vi "3_AdvancedDemo_MHT3.vi"() -> ()   [LabVIEW 2010]
uses:
  Types/MH_UIThread_Cmds.ctl
  _lib/PQ/MultiHarp/MH_InitInfo.ctl
  Types/MH_UIThread_Data.ctl
  Types/MH_InputChannel.ctl
  _lib/PQ/MultiHarp/MH_RefSource.ctl
  _lib/PQ/MultiHarp/mhlib_x86_x64_UIThread.llb/MH_DllPath_global.vi
  <vilib>/Utility/error.llb/DialogType.ctl
  Types/MH_DataProcThread_QCmds.ctl
  Types/MH_DataProcThread_QData.ctl
  Types/MH_VisThread_QCmds.ctl
  Types/MH_VisThread_QData.ctl
  Types/MH_VisThread_Data.ctl
  _lib/PQ/MultiHarp/MH_LibVersion_global.vi
  _lib/PQ/MultiHarp/MH_MeasMode.ctl
  Types/MH_SetInpChanData.ctl
  Types/MH_SetInpChanCmds.ctl
panel:
  in  "Settings":bool=TRUE
  in  "Run continuously":bool caption="Conti."
  in  "Start":bool
  in  "Scale":bool
  out "CountRates":i32[](graph)
  in  "AllChannels":T1={"Enable"=TRUE, "Offset"=0, "Level"=-100, "Edge"=0, "DeadTime"=1000, "UseDeadTime"=FALSE, "SetEnableAllChan"=TRUE, "SetEdgeAllChan"=TRUE, "SetLevelAllChan"=TRUE, "SetOffsetAllChan"=TRUE, "SetUseDTAllChan"=TRUE, "SetDeadTAllChan"=TRUE} {"DeadTime" min=800 max=160000 step=1; "Edge" items=["falling", "rising"]; "Offset" min=-100000 max=100000 step=80; "Level" min=-1200 max=1200 step=1}
  in  "HistoAcqTime":dbl=1.0 caption="Hist.Int.Time  s" min=0.1 max=360000.0 step=0.1
  in  "AcqTime":i32=360000000 caption="T3Acqu.       ms" min=1 max=360000 step=1
  in  "Binning":i32(ring) caption="Resol.            ps" items=["80", "160", "320", "640", "1280", "2560", "5120", "10240", "20480", "40960", "81920", "163840", "327680", "655360", "1310720", "2621440", "5242880", "10485760", "20971520", "41943040", "83886080", "167772160", "335544320"]
  in  "HistoOffset":i32 caption="Offset            ns" min=0 max=100000000 step=1
  out "DeltaT":dbl=6.553665536655367 caption="T.Tr.Resol.   ms" format="%.2f"
  in  "BitShift":i32=15 min=0 max=32 step=1
  in  "OvlLevel":u32=4294967295 caption="Ovl.Level" min=1024 max=65536 step=1024
  in  "StopOvl.":bool=TRUE
  out "TTraceGraph":T2(graph)={49.38852226226715, "Resolution"=0.00655367864414373, "Histogram"=[]}
  out "HistoGraph":cluster{dbl, "Resol":dbl, "Histos":u32[][]}(graph)={0.0, "Resol"=0.08, "Histos"=[]}
  in  "SyncDeadTime":i32=1000 caption="Dead T.   ps" min=800 max=160000 step=1
  in  "UseDeadTime":bool caption="Use DT."
  in  "SyncEdge":i32(ring) caption="Edge" items=["falling", "rising"]
  in  "SyncDivider":i32(ring) caption="Divider" items=["1", "2", "4", "8", "16"]
  in  "SyncOffset":i32 caption="Offset      ps" min=-100000 max=100000 step=80
  in  "SyncLevel":i32=-100 caption="Level      mV" min=-1200 max=1200 step=1
  in  "Channels":T3[](array[typedef])=[{"Name"="Inp.Chan 1", "Enable"=TRUE, "Edge"=0, "Level"=-100, "Offset"=0, "UseDeadTime"=FALSE, "DeadTime"=1000}, {"Name"="Inp.Chan 2", "Enable"=TRUE, "Edge"=0, "Level"=-100, "Offset"=0, "UseDeadTime"=FALSE, "DeadTime"=1000}, {"Name"="Inp.Chan 3", "Enable"=TRUE, "Edge"=0, "Level"=-100, "Offset"=0, "UseDeadTime"=FALSE, "DeadTime"=1000}, {"Name"="Inp.Chan 4", "Enable"=TRUE, "Edge"=0, "Level"=-100, "Offset"=0, "UseDeadTime"=FALSE, "DeadTime"=1000}, {"Name"="Inp.Chan 5", "Enable"=TRUE, "Edge"=0, "Level"=-100, "Offset"=0, "UseDeadTime"=FALSE, "DeadTime"=1000}, {"Name"="Inp.Chan 6", "Enable"=TRUE, "Edge"=0, "Level"=-100, "Offset"=0, "UseDeadTime"=FALSE, "DeadTime"=1000}, {"Name"="Inp.Chan 7", "Enable"=TRUE, "Edge"=0, "Level"=-100, "Offset"=0, "UseDeadTime"=FALSE, "DeadTime"=1000}, {"Name"="Inp.Chan 8", "Enable"=TRUE, "Edge"=0, "Level"=-100, "Offset"=0, "UseDeadTime"=FALSE, "DeadTime"=1000}, {"Name"="Inp.Chan 9", "Enable"=TRUE, "Edge"=0, "Level"=-100, "Offset"=0, "UseDeadTime"=FALSE, "DeadTime"=1000}, {"Name"="Inp.Chan 10", "Enable"=TRUE, "Edge"=0, "Level"=-100, "Offset"=0, "UseDeadTime"=FALSE, "DeadTime"=1000}, {"Name"="Inp.Chan 11", "Enable"=TRUE, "Edge"=0, "Level"=-100, "Offset"=0, "UseDeadTime"=FALSE, "DeadTime"=1000}, {"Name"="Inp.Chan 12", "Enable"=TRUE, "Edge"=0, "Level"=-100, "Offset"=0, "UseDeadTime"=FALSE, "DeadTime"=1000}, {"Name"="Inp.Chan 13", "Enable"=TRUE, "Edge"=0, "Level"=-100, "Offset"=0, "UseDeadTime"=FALSE, "DeadTime"=1000}, {"Name"="Inp.Chan 14", "Enable"=TRUE, "Edge"=0, "Level"=-100, "Offset"=0, "UseDeadTime"=FALSE, "DeadTime"=1000}, {"Name"="Inp.Chan 15", "Enable"=TRUE, "Edge"=0, "Level"=-100, "Offset"=0, "UseDeadTime"=FALSE, "DeadTime"=1000}, {"Name"="Inp.Chan 16", "Enable"=TRUE, "Edge"=0, "Level"=-100, "Offset"=0, "UseDeadTime"=FALSE, "DeadTime"=1000}] {"DeadTime" min=800 max=160000 step=1; "Edge" items=["falling", "rising"]; "Offset" min=-100000 max=100000 step=80; "Level" min=-1200 max=1200 step=1}
  out "SyncRate":string="Sync Rate: 4999940 cps\n"
  out "OverRun":bool caption="Overrun:"
  out "Status":string="Elements in Q: 0"
  # "All Channels"
  # "Acquisition"
  # "Sync"
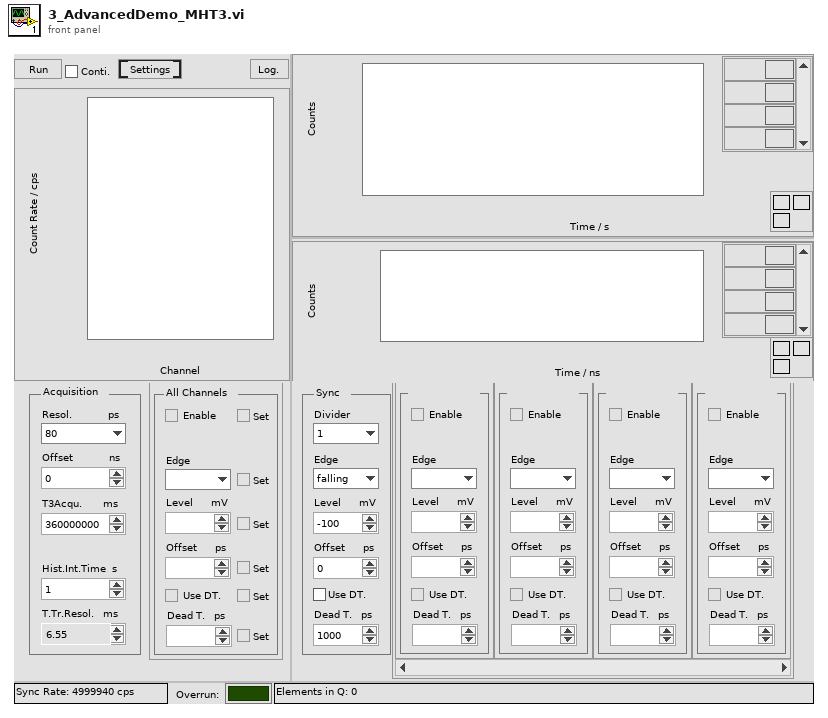
[diagram p1: front panel]
types:
  T1 = cluster{"Enable":bool, "Offset":i32, "Level":i32, "Edge":i32, "DeadTime":i32, "UseDeadTime":bool, "SetEnableAllChan":bool, "SetEdgeAllChan":bool, "SetLevelAllChan":bool, "SetOffsetAllChan":bool, "SetUseDTAllChan":bool, "SetDeadTAllChan":bool}
  T2 = cluster{dbl, "Resolution":dbl, "Histogram":u32[][]}
  T3 = typedef "MH_InputChannel.ctl" = cluster{"Name":string, "Enable":bool, "Edge":i32, "Level":i32, "Offset":i32, "UseDeadTime":bool, "DeadTime":i32}
  T4 = typedef "MH_DataProcThread_QCmds.ctl" = enum16{"Exit", "Proc", "Init", "SetShift", "SetNumChannels", "SetHistAcqTime"}
  T5 = typedef "MH_VisThread_Data.ctl" = cluster{"Resol":dbl, "DeltaT":dbl, "NumChannels":i32}
  T6 = typedef "MH_VisThread_QData.ctl" = cluster{"Histos":u32[][], "Cmd":T7, "TimeTrace":u32[][], "Bin":i32, "Total bin":u64, "Status":string, "Resol":dbl, "DeltaT":dbl, "nChannels":i32}
  T7 = typedef "MH_VisThread_QCmds.ctl" = enum16{"_none_", "Resol", "nChannels", "DeltaT", "Histo", "TTrace", "Status"}
  T8 = typedef "MH_DataProcThread_QData.ctl" = cluster{"Cmd":T4, "nActual":i32, "Buffer":u32[], "TickCount":u32, "Param":i32}
  T9 = typedef "MH_UIThread_Data.ctl" = cluster{"Init Info":T10, "DevIdx":i32, "SyncDivider":i32, "SyncOffset":i32, "SyncLevel":i32, "Channels":T3[], "CurrentChannels":i32[], "AcqTime":i32, "Binning":i32, "HistoOffset":i32, "HistoLen":i32, "StopOvl.":bool, "OvlLevel":u32, "SyncEdge":i32, "StartMeas":bool, "HistoLength":i32, "Resolution":dbl, "Run cont.":bool, "Status":string, "SyncRate":i32, "BitShift":i32, "HistoAcqTime":dbl, "SyncRateStart":i32, "UseDeadTime":bool, "SyncDeadTime":i32, "SetInpChan":T11[]}
  T10 = typedef "MH_InitInfo.ctl" = cluster{"Library Version":string, "Serial No.":string, "Model":string, "Partnum":string, "Version":string, "features":i32, "nchannels":i32, "Base Resolution":dbl, "Bin Steps":i32}
  T11 = typedef "MH_SetInpChanData.ctl" = cluster{"Channel":i32, "Cmds":T12[], "Changed":cluster{"Name":bool, "Enable":bool, "Edge":bool, "Level":bool, "Offset":bool, "UseDeadTime":bool, "DeadTime":bool}}
  T12 = typedef "MH_SetInpChanCmds.ctl" = enum16{"SetInpChanEnable", "SetInpChanOffset", "SetInpChanDeadTime", "SetInpChanTrg"}
  T13 = typedef "MH_UIThread_Cmds.ctl" = enum16{"Idle", "Init", "SetInpChan", "SetSyncDivider", "SetSyncTrg", "SetSyncOffset", "SetSyncDeadTime", "SetBinning", "SetHistoOffset", "SetHistoLen", "SetStopOvl", "SetBitShift", "SetHistoAcqTime", "GetRates", "GetAllRates", "StartMeas", "StopMeas", "AbortMeas", "GetResolution", "GetHistos", "GetAllHistos", "ReadFiFo", "WriteStatus", "Resize", "EnableControls", "DisableControls", "Error", "Exit"}
  T14 = enum8{"Enabled", "Disabled", "Disabled and Grayed Out"}
  T15 = cluster{"[0]":bool, "[1]":bool, "[2]":bool, "[3]":bool, "[4]":bool, "[5]":bool}
  T16 = typedef "MH_MeasMode.ctl" = i32
  T17 = typedef "MH_RefSource.ctl" = enum16{"INTERNAL", "EXTERNAL_10MHZ", "WR_MASTER_GENERIC", "WR_SLAVE_GENERIC", "WR_GRANDM_GENERIC", "EXTN_GPS_PPS", "EXTN_GPS_PPS_UART", "WR_MASTER_MHARP", "WR_SLAVE_MHARP", "WR_GRANDM_MHARP"}
  T18 = typedef "DialogType.ctl" = u16
  T19 = cluster{"T0":dbl, "dt":dbl, "TimeTrace_out":u32[][]}
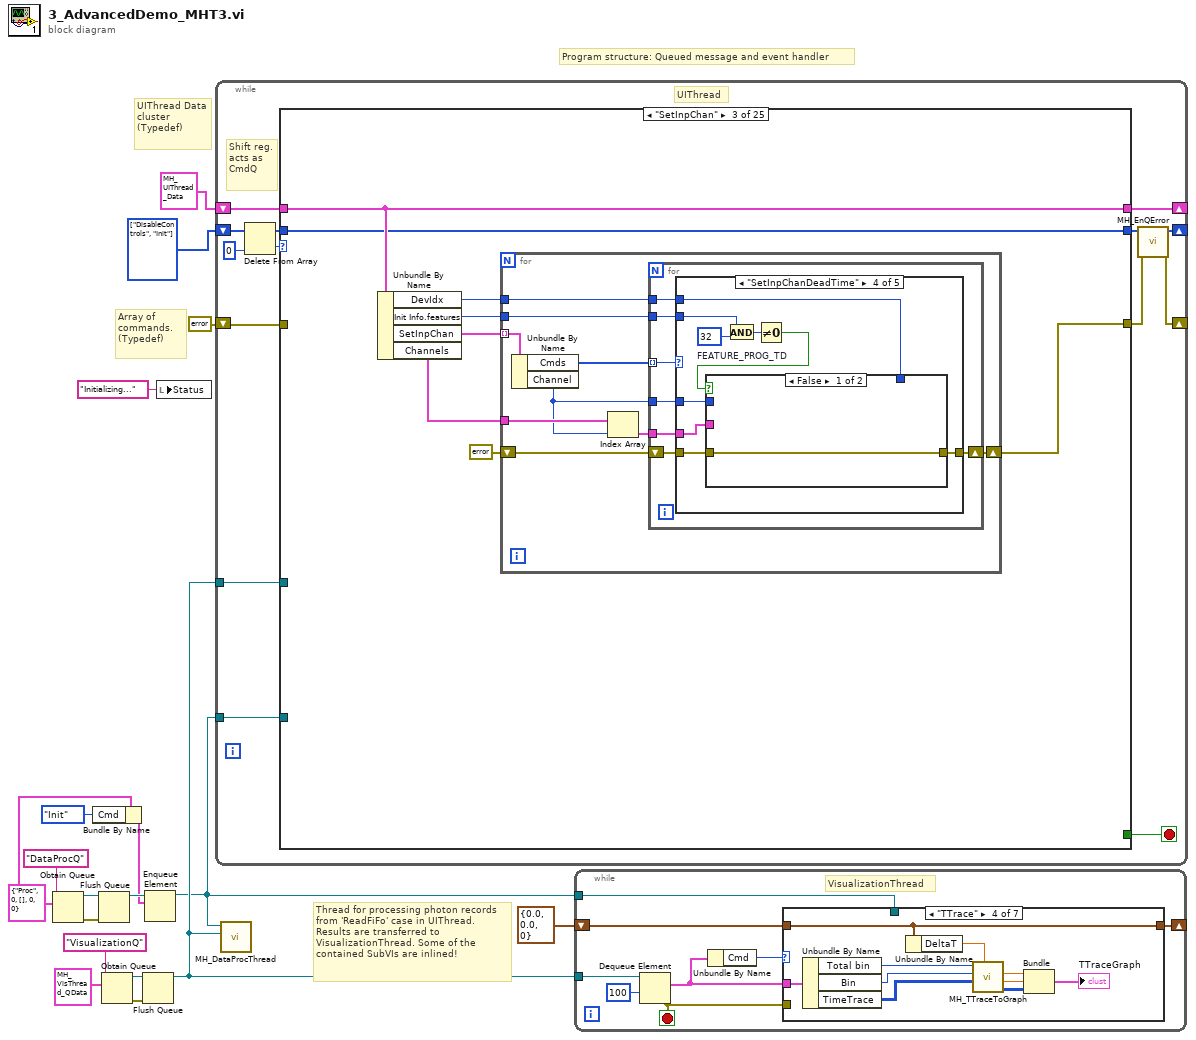
[diagram p0: block diagram]
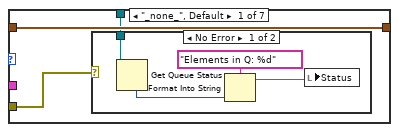
[diagram p2: hidden frame]
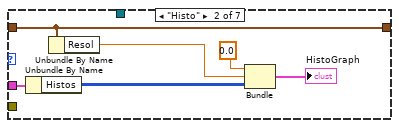
[diagram p4: hidden frame]
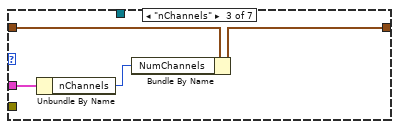
[diagram p5: hidden frame]
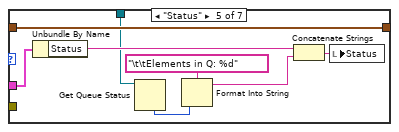
[diagram p6: hidden frame]
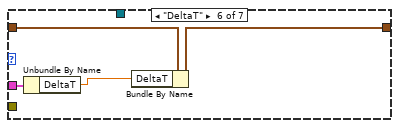
[diagram p7: hidden frame]
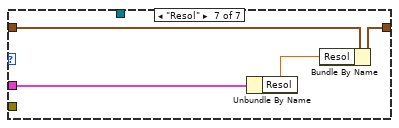
[diagram p8: hidden frame]
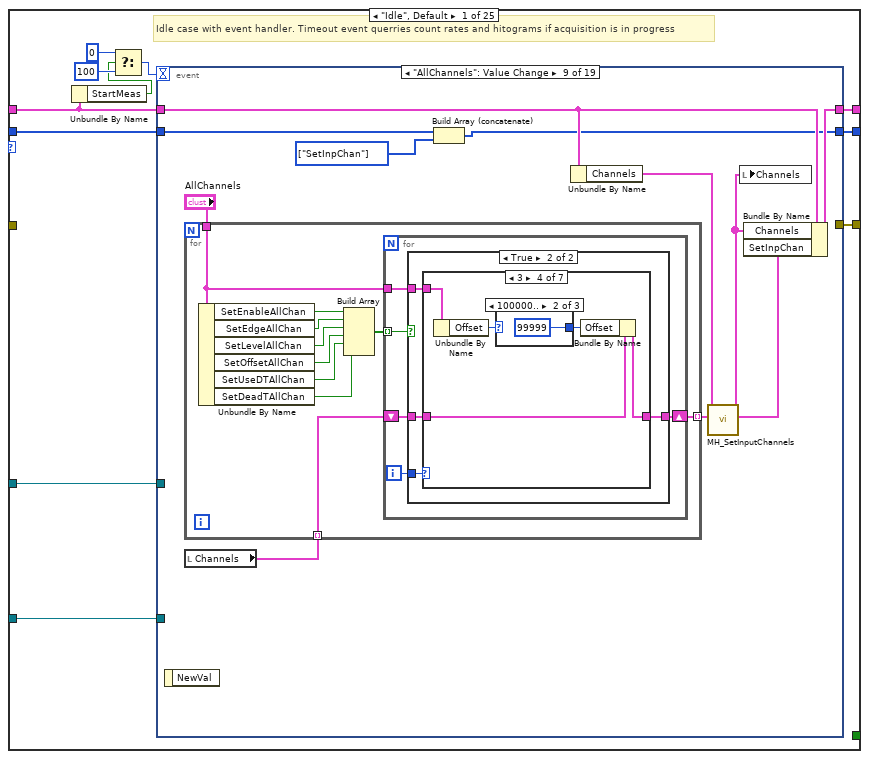
[diagram p9: hidden frame]
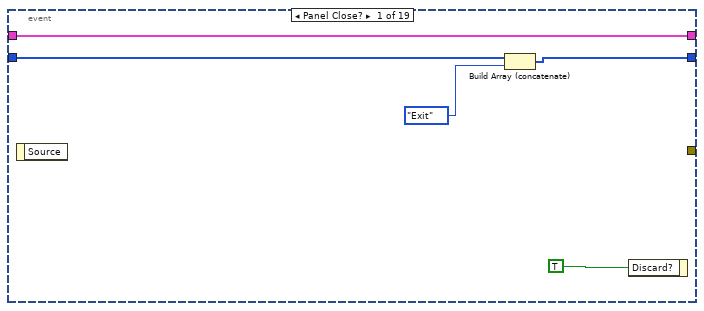
[diagram p10: hidden frame]
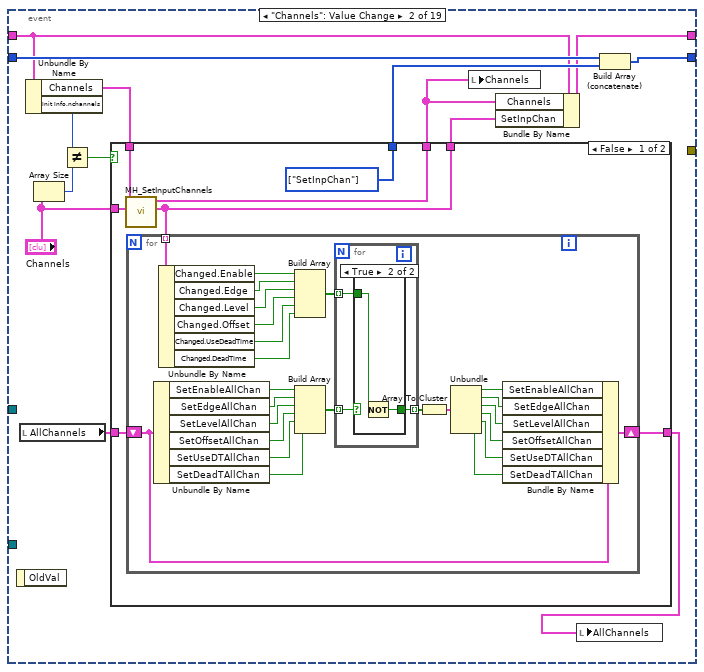
[diagram p11: hidden frame]
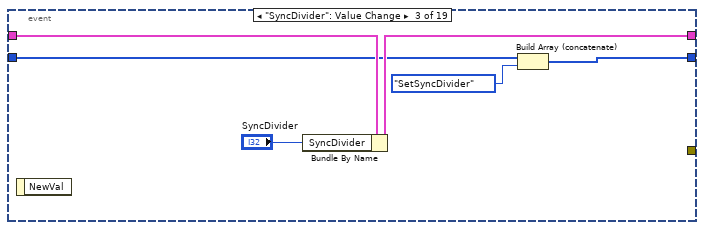
[diagram p14: hidden frame]
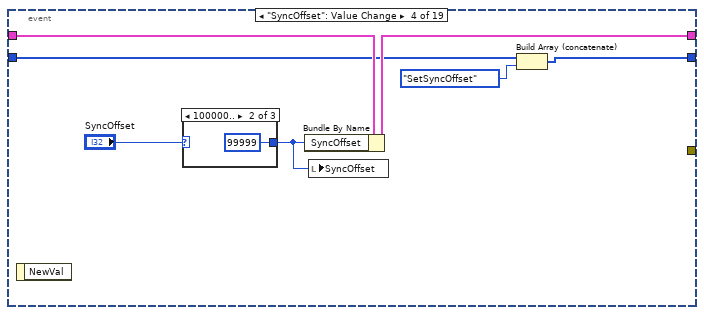
[diagram p15: hidden frame]
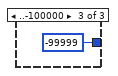
[diagram p17: hidden frame]
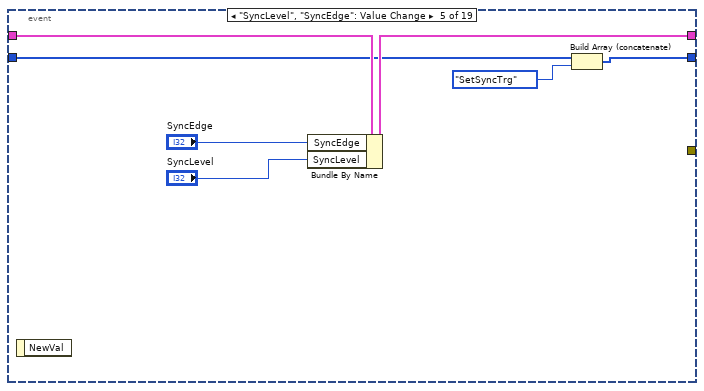
[diagram p18: hidden frame]
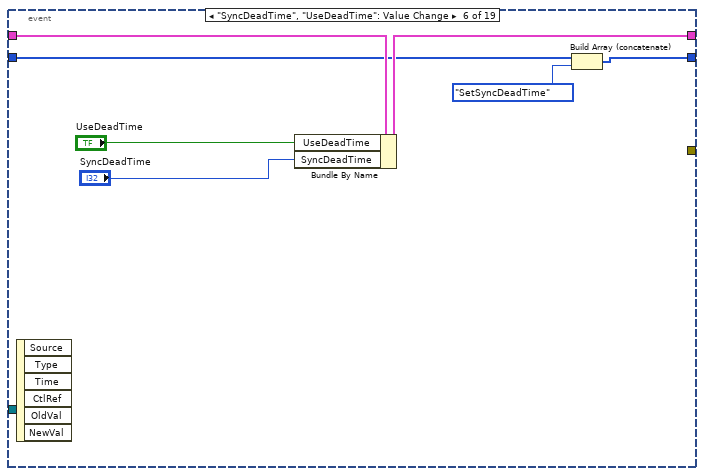
[diagram p19: hidden frame]
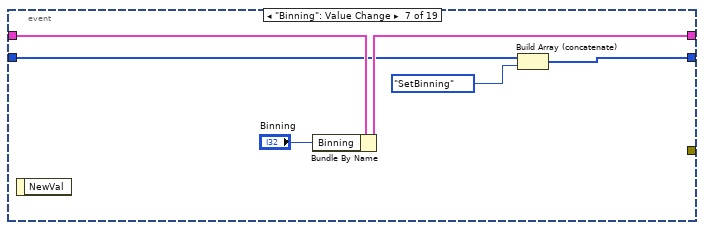
[diagram p20: hidden frame]
diagram:
  w4 = T8 {"Cmd"=enum."Proc", "nActual"=0, "Buffer"=[], "TickCount"=0, "Param"=0} ("MH_DataProcThread_QData")
  w17 = T13[] [enum."DisableControls", enum."Init"] items=["Idle", "Init", "SetInpChan", "SetSyncDivider", "SetSyncTrg", "SetSyncOffset", "SetSyncDeadTime", "SetBinning", "SetHistoOffset", "SetHistoLen", "SetStopOvl", "SetBitShift", "SetHistoAcqTime", "GetRates", "GetAllRates", "StartMeas", "StopMeas", "AbortMeas", "GetResolution", "GetHistos", "GetAllHistos", "ReadFiFo", "WriteStatus", "Resize", "EnableControls", "DisableControls", "Error", "Exit"]
  # "Thread for processing photon records from 'ReadFiFo' case in UIThread. Results are transferred to VisualizationThread. Some of the contained SubVIs are inlined!"
  # "Array of commands.\n(Typedef)"
  # "Program structure: Queued message and event handler"
  # "UIThread Data cluster\n(Typedef)"
  n1 = Obtain Queue(name (unnamed)="DataProcQ", element data type=w4) -> (queue out=w14:refnum<queue>, error out=w13:errorcluster)  [unwired: 3 in, 1 out]
  n2 = Bundle By Name(cluster=w4, "Cmd"=MH_DataProcThread_QCmds."Init") -> (w2:T8)
  n3 = Flush Queue(queue=w14, error in (no error)=w13) -> (queue out=w5:refnum<queue>)  [unwired: 2 out]
  n4 = Obtain Queue(name (unnamed)="VisualizationQ", element data type=T6 {"Histos"=[], "Cmd"=enum."_none_", "TimeTrace"=[], "Bin"=0, "Total bin"=0, "Status"="", "Resol"=0.0, "DeltaT"=0.0, "nChannels"=0} ("MH_GUIThread_QData")) -> (queue out=w12:refnum<queue>, error out=w11:errorcluster)  [unwired: 3 in, 1 out]
  n5 = Flush Queue(queue=w12, error in (no error)=w11) -> (queue out=w7:refnum<queue>)  [unwired: 2 out]
  n6 = Enqueue Element(queue=w5, element=w2) -> (queue out=w1:refnum<queue>)  [unwired: 2 in, 2 out]
  n7 = local write "Status"("Initializing..." ("Status")) -> ()
  n8 = while {
    shift-right: [w21] -> _
    shift-left: w17 -> [w28]
    shift-right: [w31] -> _
    shift-left: T9 {"Init Info"={"Library Version"="", "Serial No."="", "Model"="", "Partnum"="", "Version"="", "features"=0, "nchannels"=0, "Base Resolution"=0.0, "Bin Steps"=0}, "DevIdx"=0, "SyncDivider"=1, "SyncOffset"=0, "SyncLevel"=50, "Channels"=[], "CurrentChannels"=[], "AcqTime"=1, "Binning"=1, "HistoOffset"=1, "HistoLen"=1024, "StopOvl."=FALSE, "OvlLevel"=1024, "SyncEdge"=10, "StartMeas"=FALSE, "HistoLength"=0, "Resolution"=0.0, "Run cont."=FALSE, "Status"="", "SyncRate"=0, "BitShift"=0, "HistoAcqTime"=0.0, "SyncRateStart"=0, "UseDeadTime"=FALSE, "SyncDeadTime"=800, "SetInpChan"=[]} -> [w30]
    shift-right: [w23] -> _
    shift-left: errorcluster {"status"=FALSE, "code"=0, "source"=""} ("error IO") -> [w29]
    tunnel: w1 -> [w20]
    tunnel: w7 -> [w19]
    stop <- w32 stop-if-true
    # "Shift reg.\nacts as\nCmdQ"
    # "UIThread"
    n9 = Delete From Array(array=w28, index=0) -> (deleted portion=w26:T13, array with subset deleted=w25:T13[])  [unwired: 1 in]
    n10 = case shown="\"SetInpChan\"" w26 {
      tunnel: [w43 w357 w375 w437 w446 w458 w464 w471 w479 w486 w506 w518 w521 w593 w616 w621 w634 w651 w652 w678 w691 w698 w710 w716 w722] -> w22
      tunnel: [_ _ _ _ _ _ _ _ _ _ _ _ _ _ _ _ _ _ _ _ _ _ _ _ TRUE] -> w32
      tunnel: [w42 w338 w376 w439 w447 w459 w468 w475 w480 w487 w491 w508 w530 w585 w608 w624 w636 w647 w662 w677 w679 w697 w709 w717 w725] -> w31
      tunnel: w30 -> [w39 w343 w376 w439 w447 w459 w468 w475 w480 w487 w491 w508 w520 w586 w609 w625 w637 w648 w662 w677 w679 w697 w709 w717 w725]
      tunnel: [w40 w360 w370 w435 w445 w457 w467 w474 w478 w485 _ _ w526 w592 w619 w627 w639 w649 w657 _ _ _ _ _ w723] -> w24
      tunnel: w29 -> [_ _ _ _ _ _ _ _ _ _ _ _ _ _ _ _ _ _ _ _ _ _ _ w718 _]
      tunnel: w25 -> [w41 w359 w375 w437 w446 w458 w464 w470 w479 w486 w506 w518 w522 w593 w617 w622 w634 w651 w653 w678 w691 w698 w710 _ w722]
      tunnel: w20 -> [w34 w336 _ _ _ _ _ _ _ _ w492 w509 _ _ w613 _ _ _ w654 _ _ _ _ _ w721]
      tunnel: w19 -> [w33 w329 _ _ _ _ _ _ _ _ w493 _ _ _ _ _ _ w644 _ _ _ _ _ _ w720]
      frame "Idle", Default {
        # "Idle case with event handler. Timeout event querries count rates and hitograms if acquisition is in progress"
        n11 = Unbundle By Name(w39) -> ("StartMeas"=w37:bool)
        n12 = Select(t=0, s=w37, f=100) -> (s? t:f=w36:i32)
        n13 = event shown="[8] \"AllChannels\": Value Change" {
          selector: _ -> [_ _ _ _ _ _ _ _ _ _ _ _ _ _ _ _ _ _ _]
          dyn-events: _ -> [_ _ _ _ _ _ _ _ _ _ _ _ _ _ _ _ _ _ _]
          timeout: w36 -> [_ _ _ _ _ _ _ _ _ _ _ _ _ _ _ _ _ _ _]
          tunnel: [w44 w61 w103 w111 w120 w128 w134 w140 w145 w205 w210 w217 w232 w250 w262 w280 w286 w294 w304] -> w43
          tunnel: [w47 w53 w107 w114 w124 w131 w137 w143 w150 w207 w213 w220 w231 w254 w261 w278 w285 w293 w307] -> w42
          tunnel: w39 -> [w47 w54 w108 w115 w125 w132 w138 w144 w151 w208 w214 w221 w231 w255 w259 w279 w285 w293 w307]
          tunnel: w41 -> [w46 w62 w105 w113 w122 w130 w136 w142 w146 w205 w211 w219 w233 w251 w263 w280 w286 w294 w305]
          tunnel: [_ _ _ _ _ _ _ _ _ _ _ _ w227 _ _ _ _ _ _] -> w40
          tunnel: w34 -> [_ _ _ _ _ _ _ _ _ _ _ _ _ _ _ _ _ _ _]
          tunnel: w33 -> [_ _ _ _ _ _ _ _ _ _ _ _ _ _ _ _ _ _ _]
          event Panel Close? {
            n14 = event-data() -> ()  [unwired: 1 in, 1 out]
            n15 = Build Array (concatenate)(w46, MH_UIThread_Cmds."Exit") -> (w44:T13[])
            n16 = event-data("Discard?"=TRUE) -> ()  [unwired: 1 in, 1 out]
          }
          event "Channels": Value Change {
            n17 = event-data() -> ()  [unwired: 1 in, 1 out]
            n18 = local read "AllChannels"() -> (w49:T1)
            n19 = Unbundle By Name(w54) -> ("Channels"=w56:T3[], "Init Info.nchannels"=w58:i32)
            n20 = Array Size(array="Channels") -> (size(s)=w59:i32)
            n21 = Not Equal?(x=w58, y=w59) -> (x != y?=w57:bool)
            n22 = case shown="False" w57 {
              tunnel: "Channels" -> [w68 _]
              tunnel: [w67 w102] -> w51
              tunnel: w56 -> [w69 w102]
              tunnel: [w65 _] -> w52
              tunnel: [w66 _] -> w55
              tunnel: w49 -> [w64 w101]
              tunnel: [w63 w101] -> w50
              frame False {
                w66 = T13[] [enum."SetInpChan"] items=["Idle", "Init", "SetInpChan", "SetSyncDivider", "SetSyncTrg", "SetSyncOffset", "SetSyncDeadTime", "SetBinning", "SetHistoOffset", "SetHistoLen", "SetStopOvl", "SetBitShift", "SetHistoAcqTime", "GetRates", "GetAllRates", "StartMeas", "StopMeas", "AbortMeas", "GetResolution", "GetHistos", "GetAllHistos", "ReadFiFo", "WriteStatus", "Resize", "EnableControls", "DisableControls", "Error", "Exit"] ("array")
                n23 = call "MH_SetInputChannels.vi"("Channels new"=w68, "Channels old"=w69) -> ("SetInpChan"=w65:T11[], "Channels"=w67:T3[])  [unwired: 8 in]
                n24 = for {
                  tunnel: w65 -> [w94] mode=indexing
                  shift-right: [w76] -> w63
                  shift-left: w64 -> [w78]
                  n25 = Unbundle By Name(w78) -> ("SetEnableAllChan"=w87:bool, "SetEdgeAllChan"=w86:bool, "SetLevelAllChan"=w85:bool, "SetOffsetAllChan"=w84:bool, "SetUseDTAllChan"=w83:bool, "SetDeadTAllChan"=w82:bool)
                  n26 = Unbundle By Name(w94) -> ("Changed.Enable"=w93:bool, "Changed.Edge"=w92:bool, "Changed.Level"=w91:bool, "Changed.Offset"=w90:bool, "Changed.UseDeadTime"=w89:bool, "Changed.DeadTime"=w88:bool)
                  n27 = Build Array(w93, w92, w91, w90, w89, w88) -> (w80:bool[])
                  n28 = Build Array(w87, w86, w85, w84, w83, w82) -> (w81:bool[])
                  n29 = for {
                    tunnel: w81 -> [w97] mode=indexing
                    tunnel: w80 -> [w95] mode=indexing
                    tunnel: [w96] -> w79 mode=indexing
                    n30 = case shown="True" w97 {
                      selector: w97 -> [w98 _]
                      tunnel: [w98 w99] -> w96
                      tunnel: w95 -> [_ w100]
                      frame False {
                      }
                      frame True {
                        n31 = Not(x=w100) -> (.not. x?=w99:bool)
                      }
                    }
                  }
                  n32 = Array To Cluster(array=w79) -> (cluster=w77:T15)
                  n33 = Unbundle(w77) -> ("[0]"=w75:bool, "[1]"=w74:bool, "[2]"=w73:bool, "[3]"=w72:bool, "[4]"=w71:bool, "[5]"=w70:bool)
                  n34 = Bundle By Name(cluster=w78, "SetEnableAllChan"=w75, "SetEdgeAllChan"=w74, "SetLevelAllChan"=w73, "SetOffsetAllChan"=w72, "SetUseDTAllChan"=w71, "SetDeadTAllChan"=w70) -> (w76:T1)
                }
              }
              frame True {
              }
            }
            n35 = local write "Channels"(w51) -> ()
            n36 = Bundle By Name(cluster=w54, "Channels"=w51, "SetInpChan"=w52) -> (w53:T9)
            n37 = local write "AllChannels"(w50) -> ()
            n38 = Build Array (concatenate)(w62, w55) -> (w61:T13[])
          }
          event "SyncDivider": Value Change {
            n39 = event-data() -> ()  [unwired: 1 in, 1 out]
            n40 = Bundle By Name(cluster=w108, "SyncDivider"="SyncDivider") -> (w107:T9)
            n41 = Build Array (concatenate)(w105, MH_UIThread_Cmds."SetSyncDivider") -> (w103:T13[])
          }
          event "SyncOffset": Value Change {
            n42 = event-data() -> ()  [unwired: 1 in, 1 out]
            n43 = case shown="100000.." "SyncOffset" {
              selector: "SyncOffset" -> [w116 _ _]
              tunnel: [w116 99999 ("SyncOffset") -99999 ("SyncOffset")] -> w109
              frame Default {
              }
              frame 100000.. {
              }
              frame ..-100000 {
              }
            }
            n44 = Bundle By Name(cluster=w115, "SyncOffset"=w109) -> (w114:T9)
            n45 = local write "SyncOffset"(w109) -> ()
            n46 = Build Array (concatenate)(w113, MH_UIThread_Cmds."SetSyncOffset") -> (w111:T13[])
          }
          event "SyncLevel", "SyncEdge": Value Change {
            n47 = event-data() -> ()  [unwired: 1 in, 1 out]
            n48 = Bundle By Name(cluster=w125, "SyncEdge"="SyncEdge", "SyncLevel"="SyncLevel") -> (w124:T9)
            n49 = Build Array (concatenate)(w122, MH_UIThread_Cmds."SetSyncTrg") -> (w120:T13[])
          }
          event "SyncDeadTime", "UseDeadTime": Value Change {
            n50 = event-data() -> ()  [unwired: 1 in, 6 out]
            n51 = Bundle By Name(cluster=w132, "UseDeadTime"="UseDeadTime", "SyncDeadTime"="SyncDeadTime") -> (w131:T9)
            n52 = Build Array (concatenate)(w130, MH_UIThread_Cmds."SetSyncDeadTime") -> (w128:T13[])
          }
          event "Binning": Value Change {
            n53 = event-data() -> ()  [unwired: 1 in, 1 out]
            n54 = Bundle By Name(cluster=w138, "Binning"="Binning") -> (w137:T9)
            n55 = Build Array (concatenate)(w136, MH_UIThread_Cmds."SetBinning") -> (w134:T13[])
          }
          event "HistoOffset": Value Change {
            n56 = event-data() -> ()  [unwired: 1 in, 1 out]
            n57 = Bundle By Name(cluster=w144, "HistoOffset"="HistoOffset") -> (w143:T9)
            n58 = Build Array (concatenate)(w142, MH_UIThread_Cmds."SetHistoOffset") -> (w140:T13[])
          }
          event "AllChannels": Value Change {
            w147 = T13[] [enum."SetInpChan"] items=["Idle", "Init", "SetInpChan", "SetSyncDivider", "SetSyncTrg", "SetSyncOffset", "SetSyncDeadTime", "SetBinning", "SetHistoOffset", "SetHistoLen", "SetStopOvl", "SetBitShift", "SetHistoAcqTime", "GetRates", "GetAllRates", "StartMeas", "StopMeas", "AbortMeas", "GetResolution", "GetHistos", "GetAllHistos", "ReadFiFo", "WriteStatus", "Resize", "EnableControls", "DisableControls", "Error", "Exit"] ("array")
            n59 = event-data() -> ()  [unwired: 1 in, 1 out]
            n60 = local read "Channels"() -> (w154:T3[])
            n61 = for {
              tunnel: w154 -> [w158] mode=indexing
              tunnel: "AllChannels" -> [w157]
              tunnel: [w156] -> w153 mode=indexing
              n62 = Unbundle By Name(w157) -> ("SetEnableAllChan"=w159:bool, "SetEdgeAllChan"=w160:bool, "SetLevelAllChan"=w161:bool, "SetOffsetAllChan"=w162:bool, "SetUseDTAllChan"=w163:bool, "SetDeadTAllChan"=w164:bool)
              n63 = Build Array(w159, w160, w161, w162, w163, w164) -> (w165:bool[])
              n64 = for {
                tunnel: w165 -> [w170] mode=indexing
                shift-right: [w167] -> w156
                shift-left: w158 -> [w168]
                tunnel: w157 -> [w166]
                i -> [w169]
                n65 = case shown="True" w170 {
                  tunnel: w169 -> [_ w175]
                  tunnel: w166 -> [_ w174]
                  tunnel: w168 -> [w171 w173]
                  tunnel: [w171 w172] -> w167
                  frame False {
                  }
                  frame True {
                    n66 = case shown="3" w175 {
                      tunnel: w174 -> [w179 w183 w187 w192 w199 w203 _]
                      tunnel: w173 -> [w178 w182 w186 w191 w198 w202 w204]
                      tunnel: [w176 w180 w184 w190 w196 w200 w204] -> w172
                      frame 0 {
                        n67 = Unbundle By Name(w179) -> ("Enable"=w177:bool)
                        n68 = Bundle By Name(cluster=w178, "Enable"=w177) -> (w176:T3)
                      }
                      frame 1 {
                        n69 = Unbundle By Name(w183) -> ("Edge"=w181:i32)
                        n70 = Bundle By Name(cluster=w182, "Edge"=w181) -> (w180:T3)
                      }
                      frame 2 {
                        n71 = Unbundle By Name(w187) -> ("Level"=w185:i32)
                        n72 = Bundle By Name(cluster=w186, "Level"=w185) -> (w184:T3)
                      }
                      frame 3 {
                        n73 = Unbundle By Name(w192) -> ("Offset"=w189:i32)
                        n74 = case shown="100000.." w189 {
                          selector: w189 -> [w193 _ _]
                          tunnel: [w193 99999 ("SyncOffset") -99999 ("SyncOffset")] -> w188
                          frame Default {
                          }
                          frame 100000.. {
                          }
                          frame ..-100000 {
                          }
                        }
                        n75 = Bundle By Name(cluster=w191, "Offset"=w188) -> (w190:T3)
                      }
                      frame 4 {
                        n76 = Unbundle By Name(w199) -> ("UseDeadTime"=w197:bool)
                        n77 = Bundle By Name(cluster=w198, "UseDeadTime"=w197) -> (w196:T3)
                      }
                      frame 5 {
                        n78 = Unbundle By Name(w203) -> ("DeadTime"=w201:i32)
                        n79 = Bundle By Name(cluster=w202, "DeadTime"=w201) -> (w200:T3)
                      }
                      frame Default {
                      }
                    }
                  }
                }
              }
            }
            n80 = Build Array (concatenate)(w146, w147) -> (w145:T13[])
            n81 = Unbundle By Name(w151) -> ("Channels"=w152:T3[])
            n82 = call "MH_SetInputChannels.vi"("Channels new"=w153, "Channels old"=w152) -> ("SetInpChan"=w148:T11[], "Channels"=w149:T3[])  [unwired: 8 in]
            n83 = local write "Channels"(w149) -> ()
            n84 = Bundle By Name(cluster=w151, "Channels"=w149, "SetInpChan"=w148) -> (w150:T9)
          }
          event "AcqTime": Value Change {
            n85 = event-data() -> ()  [unwired: 1 in, 1 out]
            n86 = Bundle By Name(cluster=w208, "AcqTime"="AcqTime") -> (w207:T9)
          }
          event "HistoAcqTime": Value Change {
            n87 = event-data() -> ()  [unwired: 1 in, 1 out]
            n88 = Bundle By Name(cluster=w214, "HistoAcqTime"="HistoAcqTime") -> (w213:T9)
            n89 = Build Array (concatenate)(w211, MH_UIThread_Cmds."SetHistoAcqTime") -> (w210:T13[])
          }
          event "OvlLevel", "StopOvl.": Value Change {
            n90 = event-data() -> ()  [unwired: 1 in, 1 out]
            n91 = Bundle By Name(cluster=w221, "StopOvl."="StopOvl.", "OvlLevel"="OvlLevel") -> (w220:T9)
            n92 = Build Array (concatenate)(w219, MH_UIThread_Cmds."SetStopOvl") -> (w217:T13[])
          }
          event Timeout {
            n93 = event-data() -> ()  [unwired: 1 in, 1 out]
            n94 = Unbundle By Name(w231) -> ("DevIdx"=w229:i32, "StartMeas"=w230:bool, "BitShift"=w226:i32, "SyncRate"=w225:i32)
            n95 = case shown="True" w230 {
              tunnel: w229 -> [_ w249]
              tunnel: [_ w247] -> w228
              tunnel: [_ w244] -> w227
              frame False {
              }
              frame True {
                w245 = T13[] [enum."ReadFiFo"] items=["Idle", "Init", "SetInpChan", "SetSyncDivider", "SetSyncTrg", "SetSyncOffset", "SetSyncDeadTime", "SetBinning", "SetHistoOffset", "SetHistoLen", "SetStopOvl", "SetBitShift", "SetHistoAcqTime", "GetRates", "GetAllRates", "StartMeas", "StopMeas", "AbortMeas", "GetResolution", "GetHistos", "GetAllHistos", "ReadFiFo", "WriteStatus", "Resize", "EnableControls", "DisableControls", "Error", "Exit"]
                w246 = T13[] [enum."StopMeas"] items=["Idle", "Init", "SetInpChan", "SetSyncDivider", "SetSyncTrg", "SetSyncOffset", "SetSyncDeadTime", "SetBinning", "SetHistoOffset", "SetHistoLen", "SetStopOvl", "SetBitShift", "SetHistoAcqTime", "GetRates", "GetAllRates", "StartMeas", "StopMeas", "AbortMeas", "GetResolution", "GetHistos", "GetAllHistos", "ReadFiFo", "WriteStatus", "Resize", "EnableControls", "DisableControls", "Error", "Exit"]
                n96 = call "MH_CTCStatus.vi"("devidx"=w249) -> ("error out"=w244:errorcluster, "ctcstatus"=w248:i32)  [unwired: 8 in, 1 out]
                n97 = Not Equal To 0?(x=w248) -> (x != 0?=w243:bool)
                n98 = Select(t=w246, s=w243, f=w245) -> (s? t:f=w247:T13[])
              }
            }
            n99 = call "CalcRate.vi"("Refresh(ms)"=u32 100) -> ("updated?"=w223:bool)  [unwired: 8 in, 2 out]
            n100 = case shown="True" w223 {
              tunnel: w226 -> [_ w236]
              tunnel: w225 -> [_ w235]
              tunnel: [_ MH_UIThread_Cmds."GetAllRates"] -> w224
              frame False {
              }
              frame True {
                n101 = To Double Precision Float(number=w235) -> (double precision float=w240:dbl)
                n102 = To Double Precision Float(number=w236) -> (double precision float=w241:dbl)
                n103 = Power Of 2(x=w241) -> (2^x=w239:dbl)
                n104 = Multiply(x=w239, y=1000.0) -> (x*y=w238:dbl)
                n105 = Divide(x=w238, y=w240) -> (x/y=w242:dbl)
                n106 = local write "DeltaT"(w242) -> ()
              }
            }
            n107 = Build Array (concatenate)(w233, w228, w224) -> (w232:T13[])
          }
          event "BitShift": Value Change {
            n108 = event-data() -> ()  [unwired: 1 in, 1 out]
            n109 = Bundle By Name(cluster=w255, "BitShift"="BitShift") -> (w254:T9)
            n110 = Build Array (concatenate)(w251, MH_UIThread_Cmds."SetBitShift") -> (w250:T13[])
          }
          event "Start": Value Change {
            n111 = event-data() -> ()  [unwired: 1 in, 1 out]
            n112 = Unbundle By Name(w259) -> ("SyncRate"=w258:i32)
            n113 = Greater Or Equal?(x=w258, y=10) -> (x >= y?=w256:bool)
            n114 = case shown="True" w256 {
              selector: w256 -> [w265 _]
              tunnel: w263 -> [w267 w276]
              tunnel: [w267 w274] -> w262
              tunnel: [w266 w273] -> w261
              tunnel: "Start" -> [_ w272]
              tunnel: w259 -> [w266 w268]
              frame False {
                n115 = local write "Start"(w265) -> ()
                n116 = One Button Dialog(message="SyncRate too low!!!" ("Status")) -> ()  [unwired: 1 in, 1 out]
              }
              frame True {
                w271 = T13[] [enum."SetBitShift", enum."SetHistoAcqTime", enum."StartMeas"] items=["Idle", "Init", "SetInpChan", "SetSyncDivider", "SetSyncTrg", "SetSyncOffset", "SetSyncDeadTime", "SetBinning", "SetHistoOffset", "SetHistoLen", "SetStopOvl", "SetBitShift", "SetHistoAcqTime", "GetRates", "GetAllRates", "StartMeas", "StopMeas", "AbortMeas", "GetResolution", "GetHistos", "GetAllHistos", "ReadFiFo", "WriteStatus", "Resize", "EnableControls", "DisableControls", "Error", "Exit"]
                n117 = Bundle By Name(cluster=w268, "StartMeas"=w272) -> (w273:T9)
                n118 = Build Array(MH_UIThread_Cmds."AbortMeas") -> (w269:T13[])
                n119 = Select(t=w271, s=w272, f=w269) -> (s? t:f=w275:T13[])
                n120 = Build Array (concatenate)(w276, w275) -> (w274:T13[])
              }
            }
          }
          event "Run continuously": Value Change {
            n121 = event-data() -> ()  [unwired: 1 in, 1 out]
            n122 = Bundle By Name(cluster=w279, "Run cont."="Run continuously") -> (w278:T9)
          }
          event "Scale": Value Change {
            n123 = event-data() -> ()  [unwired: 1 in, 1 out]
            n124 = Select(t=u8 0 ("Y Scale.Mapping Mode"), s="Scale", f=u8 1 ("Y Scale.Mapping Mode")) -> (s? t:f=w281:u8)
            n125 = property on="HistoGraph" class="WFGraph (strict)"("YScale.Mapping Mode"=w281) -> ()  [unwired: 2 in, 2 out]
          }
          event "Settings": Value Change {
            n126 = event-data() -> ()  [unwired: 1 in, 1 out]
            n127 = property on="Splitter" class="Splitter"() -> ("Position"=w292:i32)  [unwired: 2 in, 2 out]
            n128 = Select(t=300 ("PosT"), s="Settings", f=0 ("PosF")) -> (s? t:f=w289:i32)
            n129 = Subtract(x=w292, y=w289) -> (x-y=w288:i32)
            n130 = while {
              shift-right: [w303] -> _
              shift-left: w288 -> [w296]
              i -> [w302]
              stop <- w299 stop-if-true
              n131 = property on="Splitter 4" class="Splitter"("Position"=w296) -> (error out=w295:errorcluster)  [unwired: 2 in, 1 out]
              n132 = Greater Or Equal?(x=w302, y=10) -> (x >= y?=w300:bool)
              n133 = Decrement(x=w296) -> (x-1=w303:i32)
              n134 = Unbundle(w295) -> ("status"=w298:bool)  [unwired: 2 out]
              n135 = Not(x=w298) -> (.not. x?=w297:bool)
              n136 = Or(x=w297, y=w300) -> (x .or. y?=w299:bool)
            }
          }
          event Panel Resize {
            n137 = event-data() -> ()  [unwired: 1 in, 1 out]
            n138 = Build Array (concatenate)(w305, MH_UIThread_Cmds."Resize") -> (w304:T13[])
          }
        }
      }
      frame "Init" {
        w316 = 1000 ("SyncDeadTime")
        w317 = FALSE ("UseDeadTime")
        w319 = T16 3 items=["HIST"=0, "T2"=2, "T3"=3]  # Mode
        w321 = MH_RefSource."INTERNAL"  # refsource
        w327 = 1.0 ("HistoAcqTime")
        w328 = 15 ("Value (Signaling)")
        w345 = FALSE ("Run cont.")
        w347 = FALSE ("StartMeas")
        w348 = u32 4294967295 ("OvlLevel")
        w349 = TRUE ("StopOvl.")
        w350 = 360000000 ("AcqTime")
        w351 = 0 ("HistoOffset")
        w352 = 0 ("Binning")
        w353 = -100 ("SyncLevel")
        w354 = 0 ("SyncZeroX")
        w355 = 0 ("SyncOffset")
        w356 = 0 ("SyncDivider")
        w358 = T13[] [enum."SetSyncDivider", enum."SetSyncOffset", enum."SetSyncDeadTime", enum."SetSyncTrg", enum."SetInpChan", enum."SetBinning", enum."SetHistoOffset", enum."Resize", enum."EnableControls", enum."GetRates", enum."SetBitShift", enum."SetHistoAcqTime", enum."WriteStatus"] items=["Idle", "Init", "SetInpChan", "SetSyncDivider", "SetSyncTrg", "SetSyncOffset", "SetSyncDeadTime", "SetBinning", "SetHistoOffset", "SetHistoLen", "SetStopOvl", "SetBitShift", "SetHistoAcqTime", "GetRates", "GetAllRates", "StartMeas", "StopMeas", "AbortMeas", "GetResolution", "GetHistos", "GetAllHistos", "ReadFiFo", "WriteStatus", "Resize", "EnableControls", "DisableControls", "Error", "Exit"]
        # "100 x 60 x 60 x 1000 = 100 h"
        # "Init all FP controls and corresponding copy in UIThread Data cluster"
        # "EnQ list of commands"
        # "Array with Inp.Chan."
        # "Initialization: 1. Init HW -> get # of channels -> make array for Inp.Channels\n2. Init all FP controls and corresponding fields in UIThread Data cluster\n3. EnQ list of commands for further initialization"
        n139 = disable-structure shown="TARGET_TYPE==Windows, Default" {
          disable-tunnel: ["MHLib64" ("name or relative path") "MHLib" ("name or relative path")] -> w318
          frame condition #0 (active) {
          }
          frame condition #1 {
          }
        }
        n140 = call <vilib>:"Error Cluster From Error Code.vi"("is warning? (False)"=FALSE, "show call chain? (False)"=TRUE, "error message (\"\")"="DLL not found!" ("error message (\"\")"), "error code (0)"=5000) -> ("error out"=w322:errorcluster)  [unwired: 5 in]
        n141 = call "GetDLLPath.vi"("DllName_32bit"="MHLib" ("name or relative path"), "DllName_64bit"=w318) -> ("file exists?"=w324:bool, "DLLPath"=w325:path)  [unwired: 8 in]
        n142 = global write "MH_DllPath_global.vi" "DllPath"(w325) -> ()
        n143 = property on="AllChannels" class="Clust (strict)"("Val(Sgnl)"=T1 {"Enable"=TRUE, "Offset"=0, "Level"=-100, "Edge"=0, "DeadTime"=1000, "UseDeadTime"=FALSE, "SetEnableAllChan"=TRUE, "SetEdgeAllChan"=TRUE, "SetLevelAllChan"=TRUE, "SetOffsetAllChan"=TRUE, "SetUseDTAllChan"=TRUE, "SetDeadTAllChan"=TRUE} ("AllChannels")) -> ()  [unwired: 2 in, 2 out]
        n144 = Select(t=errorcluster {"status"=FALSE, "code"=0, "source"=""} ("error IO"), s=w324, f=w322) -> (s? t:f=w339:errorcluster)
        n145 = global read "MH_LibVersion_global.vi" "Library Version"() -> (w320:string)
        n146 = Build Array (concatenate)(w359, w358) -> (w357:T13[])
        n147 = call "InitMH_UIThread.vi"("error in (no error)"=w339, "Mode"=w319, "refsource"=w321, "Library Version"=w320) -> ("error out"=w360:errorcluster, "Init Info"=w362:T10, "DevIdx"=w361:i32)  [unwired: 5 in]
        n148 = local write "SyncDivider"(w356) -> ()
        n149 = local write "SyncOffset"(w355) -> ()
        n150 = local write "SyncEdge"(w354) -> ()
        n151 = local write "SyncLevel"(w353) -> ()
        n152 = local write "Binning"(w352) -> ()
        n153 = Bundle By Name(cluster=w343, "DevIdx"=w361, "Init Info"=w362, "Status"="Initialized!") -> (w342:T9)
        n154 = Unbundle By Name(w342) -> ("Init Info.Bin Steps"=w341:i32, "Init Info.nchannels"=w315:i32)
        n155 = for {
          N: w315 -> [_]
          i -> [w365]
          n156 = Increment(x=w365) -> (x+1=w368:i32)
          n157 = Format Into String(format string="Ch.%d", w368) -> (resulting string=w366:string)  [unwired: 2 in, 1 out]
          n158 = property on="HistoGraph" class="WFGraph (strict)"("Active Plot"=w365, "Plot.Plot Name"=w366) -> ()  [unwired: 2 in, 2 out]
          n159 = property on="TTraceGraph" class="WFGraph (strict)"("Active Plot"=w365, "Plot.Plot Name"=w366) -> ()  [unwired: 2 in, 2 out]
        }
        n160 = Bundle By Name(cluster=T6 {"Histos"=[], "Cmd"=enum."_none_", "TimeTrace"=[], "Bin"=0, "Total bin"=0, "Status"="", "Resol"=0.0, "DeltaT"=0.0, "nChannels"=0} ("MH_GUIThread_QData"), "Cmd"=MH_VisThread_QCmds."nChannels", "nChannels"=w315) -> (w331:T6)
        n161 = call "MH_CalcBinningValues.vi"("Bin Steps"=w341) -> ("BinningValues"=w346:cluster{"String":string, "Value":i32}[])  [unwired: 10 in]
        n162 = call "MH_InitChannels.vi"("nchannels"=w315) -> ("SetInpChan"=w313:T11[], "Channels"=w314:T3[])  [unwired: 9 in]
        n163 = property on="Binning" class="Ring (strict)"("StringsAndValues[]"=w346) -> ()  [unwired: 2 in, 2 out]
        n164 = Bundle By Name(cluster=T8 {"Cmd"=enum."Proc", "nActual"=0, "Buffer"=[], "TickCount"=0, "Param"=0} ("MH_DataProcThread_QData"), "Param"=w315, "Cmd"=MH_DataProcThread_QCmds."SetNumChannels") -> (w335:T8)
        n165 = Enqueue Element(queue=w329, element=w331) -> ()  [unwired: 2 in, 3 out]
        n166 = Enqueue Element(queue=w336, element=w335) -> ()  [unwired: 2 in, 3 out]
        n167 = local write "Channels"(w314) -> ()
        n168 = Bundle By Name(cluster=w342, "Channels"=w314, "SetInpChan"=w313, "SyncDivider"=w356, "SyncOffset"=w355, "SyncEdge"=w354, "SyncLevel"=w353, "Binning"=w352, "HistoOffset"=w351, "AcqTime"=w350, "StopOvl."=w349, "OvlLevel"=w348, "StartMeas"=w347, "Run cont."=w345, "BitShift"=w328, "HistoAcqTime"=w327, "UseDeadTime"=w317, "SyncDeadTime"=w316) -> (w338:T9)
        n169 = local write "AcqTime"(w350) -> ()
        n170 = local write "StopOvl."(w349) -> ()
        n171 = local write "OvlLevel"(w348) -> ()
        n172 = local write "Start"(w347) -> ()
        n173 = local write "Run continuously"(w345) -> ()
        n174 = local write "BitShift"(w328) -> ()
        n175 = local write "HistoAcqTime"(w327) -> ()
        n176 = local write "HistoOffset"(w351) -> ()
        n177 = local write "UseDeadTime"(w317) -> ()
        n178 = local write "SyncDeadTime"(w316) -> ()
        n179 = property on="Settings" class="Bool (strict)"("Val(Sgnl)"=TRUE ("Value (Signaling)")) -> ()  [unwired: 2 in, 2 out]
        n180 = property on="Scale" class="Bool (strict)"("Val(Sgnl)"=FALSE ("Value (Signaling)")) -> ()  [unwired: 2 in, 2 out]
      }
      frame "SetInpChan" {
        n181 = Unbundle By Name(w376) -> ("DevIdx"=w374:i32, "Init Info.features"=w373:i32, "SetInpChan"=w372:T11[], "Channels"=w371:T3[])
        n182 = for {
          tunnel: w371 -> [w381]
          tunnel: w372 -> [w385] mode=indexing
          shift-right: [w383] -> w370
          shift-left: errorcluster {"status"=FALSE, "code"=0, "source"=""} ("error out") -> [w382]
          tunnel: w374 -> [w379]
          tunnel: w373 -> [w377]
          n183 = Unbundle By Name(w385) -> ("Cmds"=w384:T12[], "Channel"=w378:i32)
          n184 = Index Array(array=w381, index=w378) -> (element=w380:T3)
          n185 = for {
            tunnel: w384 -> [w392] mode=indexing
            tunnel: w378 -> [w391]
            shift-right: [w390] -> w383
            shift-left: w382 -> [w389]
            tunnel: w380 -> [w388]
            tunnel: w379 -> [w387]
            tunnel: w377 -> [w386]
            n186 = case shown="\"SetInpChanDeadTime\"" w392 {
              tunnel: w391 -> [_ w398 w405 w410 w426]
              tunnel: [w393 w397 w404 w414 w431] -> w390
              tunnel: w389 -> [w393 w396 w403 w413 w430]
              tunnel: w388 -> [_ w395 w402 w412 w429]
              tunnel: w387 -> [_ w394 w401 w411 w428]
              tunnel: w386 -> [_ _ _ w407 _]
              frame Default {
              }
              frame "SetInpChanEnable" {
                n187 = Unbundle By Name(w395) -> ("Enable"=w399:bool)
                n188 = call "MH_SetInputChannelEnable.vi"("error in (no error)"=w396, "enable"=w399, "channel"=w398, "devidx"=w394) -> ("error out"=w397:errorcluster)  [unwired: 6 in, 1 out]
              }
              frame "SetInpChanOffset" {
                n189 = Unbundle By Name(w402) -> ("Offset"=w400:i32)
                n190 = call "MH_SetInputChannelOffset.vi"("error in (no error)"=w403, "Offset"=w400, "channel"=w405, "devidx"=w401) -> ("error out"=w404:errorcluster)  [unwired: 6 in, 1 out]
              }
              frame "SetInpChanDeadTime" {
                w408 = 32  # FEATURE_PROG_TD
                n191 = And(x=w407, y=w408) -> (x .and. y?=w409:i32)
                n192 = Not Equal To 0?(x=w409) -> (x != 0?=w406:bool)
                n193 = case shown="False" w406 {
                  tunnel: [w415 w424] -> w414
                  tunnel: w413 -> [w415 w423]
                  tunnel: w412 -> [_ w422]
                  tunnel: w411 -> [_ w421]
                  tunnel: w410 -> [_ w419]
                  frame False {
                  }
                  frame True {
                    n194 = Unbundle By Name(w422) -> ("UseDeadTime"=w418:bool, "DeadTime"=w420:i32)
                    n195 = Boolean To (0,1)(Boolean=w418) -> (0, 1=w417:i16)
                    n196 = To Long Integer(number=w417) -> (32bit integer=w416:i32)
                    n197 = call "MH_SetInputDeadTime.vi"("channel"=w419, "error in (no error)"=w423, "deadtime"=w420, "on"=w416, "devidx"=w421) -> ("error out"=w424:errorcluster)  [unwired: 5 in, 1 out]
                  }
                }
              }
              frame "SetInpChanTrg" {
                n198 = Unbundle By Name(w429) -> ("Level"=w425:i32, "Edge"=w427:i32)
                n199 = call "MH_SetInputEdgeTrg.vi"("channel"=w426, "error in (no error)"=w430, "edge"=w427, "level"=w425, "devidx"=w428) -> ("error out"=w431:errorcluster)  [unwired: 5 in, 1 out]
              }
            }
          }
        }
      }
      frame "SetSyncDivider" {
        n200 = Unbundle By Name(w439) -> ("DevIdx"=w438:i32, "SyncDivider"=w434:i32)
        n201 = Power Of 2(x=w434) -> (2^x=w433:dbl)
        n202 = To Long Integer(number=w433) -> (32bit integer=w432:i32)
        n203 = call "MH_SetSyncDiv.vi"("SyncDivider"=w432, "devidx"=w438) -> ("error out"=w436:errorcluster)  [unwired: 8 in, 1 out]
        n204 = flat-sequence {
          tunnel: w436 -> [w440]
          tunnel: [w440] -> w435
          frame #0 {
            n205 = Wait (ms)(milliseconds to wait=u32 100) -> ()  [unwired: 1 out]
          }
        }
      }
      frame "SetSyncTrg" {
        n206 = Unbundle By Name(w447) -> ("DevIdx"=w444:i32, "SyncLevel"=w442:i32, "SyncEdge"=w443:i32)
        n207 = call "MH_SetSyncEdgeTrg.vi"("edge"=w443, "level"=w442, "devidx"=w444) -> ("error out"=w445:errorcluster)  [unwired: 7 in, 1 out]
      }
      frame "SetSyncDeadTime" {
        w450 = 32  # FEATURE_PROG_TD
        n208 = Unbundle By Name(w459) -> ("DevIdx"=w456:i32, "UseDeadTime"=w453:bool, "SyncDeadTime"=w455:i32, "Init Info.features"=w449:i32)
        n209 = And(x=w449, y=w450) -> (x .and. y?=w451:i32)
        n210 = Boolean To (0,1)(Boolean=w453) -> (0, 1=w454:i16)
        n211 = Not Equal To 0?(x=w451) -> (x != 0?=w448:bool)
        n212 = To Long Integer(number=w454) -> (32bit integer=w452:i32)
        n213 = case shown="True" w448 {
          tunnel: [_ w463] -> w457
          tunnel: w456 -> [_ w462]
          tunnel: w455 -> [_ w461]
          tunnel: w452 -> [_ w460]
          frame False {
          }
          frame True {
            n214 = call "MH_SetSyncDeadTime.vi"("deadtime"=w461, "on"=w460, "devidx"=w462) -> ("error out"=w463:errorcluster)  [unwired: 7 in, 1 out]
          }
        }
      }
      frame "SetSyncOffset" {
        n215 = Unbundle By Name(w468) -> ("DevIdx"=w466:i32, "SyncOffset"=w465:i32)
        n216 = call "MH_SetSyncChannelOffset.vi"("Offset"=w465, "devidx"=w466) -> ("error out"=w467:errorcluster)  [unwired: 8 in, 1 out]
      }
      frame "SetBinning" {
        # "When binning is changed the new resolution is querried"
        n217 = Unbundle By Name(w475) -> ("DevIdx"=w473:i32, "Binning"=w472:i32)
        n218 = call "MH_SetBinning.vi"("Binning"=w472, "devidx"=w473) -> ("error out"=w474:errorcluster)  [unwired: 8 in, 1 out]
        n219 = Build Array (concatenate)(MH_UIThread_Cmds."GetResolution", w470) -> (w471:T13[])
      }
      frame "SetHistoOffset" {
        n220 = Unbundle By Name(w480) -> ("DevIdx"=w477:i32, "HistoOffset"=w476:i32)
        n221 = call "MH_SetOffset.vi"("Offset"=w476, "devidx"=w477) -> ("error out"=w478:errorcluster)  [unwired: 8 in, 1 out]
      }
      frame "SetStopOvl" {
        n222 = Unbundle By Name(w487) -> ("DevIdx"=w484:i32, "StopOvl."=w483:bool, "OvlLevel"=w482:u32)
        n223 = To Unsigned Long Integer(number=w482) -> (unsigned 32bit integer=w481:u32)
        n224 = call "MH_SetStopOverflow.vi"("stopcount"=w481, "StopOnOverflow"=w483, "devidx"=w484) -> ("error out"=w485:errorcluster)  [unwired: 7 in, 1 out]
      }
      frame "SetBitShift" {
        n225 = Unbundle By Name(w491) -> ("BitShift"=w489:i32, "SyncRate"=w490:i32)
        n226 = Negate(x=w489) -> (-x=w499:i32)
        n227 = Bundle By Name(cluster=T8 {"Cmd"=enum."Proc", "nActual"=0, "Buffer"=[], "TickCount"=0, "Param"=0} ("MH_DataProcThread_QData"), "Param"=w499, "Cmd"=MH_DataProcThread_QCmds."SetShift") -> (w505:T8)
        n228 = To Double Precision Float(number=w489) -> (double precision float=w504:dbl)
        n229 = To Double Precision Float(number=w490) -> (double precision float=w503:dbl)
        n230 = Power Of 2(x=w504) -> (2^x=w502:dbl)
        n231 = Enqueue Element(queue=w492, element=w505) -> ()  [unwired: 2 in, 3 out]
        n232 = Multiply(x=w502, y=1000.0) -> (x*y=w501:dbl)
        n233 = Divide(x=w501, y=w503) -> (x/y=w488:dbl)
        "DeltaT" <- w488
        n234 = Bundle By Name(cluster=T6 {"Histos"=[], "Cmd"=enum."_none_", "TimeTrace"=[], "Bin"=0, "Total bin"=0, "Status"="", "Resol"=0.0, "DeltaT"=0.0, "nChannels"=0} ("MH_GUIThread_QData"), "DeltaT"=w488, "Cmd"=MH_VisThread_QCmds."DeltaT") -> (w500:T6)
        n235 = Enqueue Element(queue=w493, element=w500) -> ()  [unwired: 2 in, 3 out]
      }
      frame "SetHistoAcqTime" {
        n236 = Unbundle By Name(w508) -> ("SyncRate"=w514:i32, "HistoAcqTime"=w507:dbl)
        n237 = To Double Precision Float(number=w514) -> (double precision float=w517:dbl)
        n238 = Multiply(x=w517, y=w507) -> (x*y=w516:dbl)
        n239 = Round To Nearest(number=w516) -> (nearest integer value=w515:dbl)
        n240 = To Long Integer(number=w515) -> (32bit integer=w513:i32)
        n241 = Bundle By Name(cluster=T8 {"Cmd"=enum."Proc", "nActual"=0, "Buffer"=[], "TickCount"=0, "Param"=0} ("MH_DataProcThread_QData"), "Param"=w513, "Cmd"=MH_DataProcThread_QCmds."SetHistAcqTime") -> (w512:T8)
        n242 = Enqueue Element(queue=w509, element=w512) -> ()  [unwired: 2 in, 3 out]
      }
      frame "GetAllRates" {
        # "An alternative to GetRates"
        n243 = Unbundle By Name(w520) -> ("DevIdx"=w528:i32, "Init Info.nchannels"=w535:i32, "StartMeas"=w529:bool, "SyncRateStart"=w523:i32)
        n244 = call "MH_AllocateCntRateBuffer.vi"("NumChan"=w535) -> ("Buffer"=w534:i32[])  [unwired: 10 in]
        n245 = call "MH_GetAllCountRates.vi"("cntrates_buf"=w534, "devidx"=w528) -> ("error out"=w527:errorcluster, "cntrates"=→"CountRates":i32[], "syncrate"=w525:i32)  [unwired: 6 in, 1 out]
        n246 = case shown="True" w529 {
          tunnel: w528 -> [_ w550]
          tunnel: w527 -> [w539 w549]
          tunnel: [w539 w548] -> w526
          tunnel: w525 -> [w538 _]
          tunnel: [w538 w545] -> w524
          tunnel: w523 -> [_ w540]
          tunnel: w522 -> [w537 w544]
          tunnel: [w537 w543] -> w521
          tunnel: w520 -> [w536 w542]
          tunnel: [w536 w541] -> w519
          frame False {
          }
          frame True {
            n247 = call "MH_GetSyncPeriod.vi"("error in (no error)"=w549, "devidx"=w550) -> ("error out"=w548:errorcluster, "period"=w547:dbl)  [unwired: 7 in, 1 out]
            n248 = Reciprocal(x=w547) -> (1/x=w546:dbl)
            n249 = To Long Integer(number=w546) -> (32bit integer=w545:i32)
            n250 = case shown="-1" w540 {
              selector: w540 -> [w551 _ _]
              tunnel: w545 -> [w554 w575 _]
              tunnel: w544 -> [w552 w577 w581]
              tunnel: [w553 w577 w581] -> w543
              tunnel: w542 -> [w558 w576 w580]
              tunnel: [w558 w574 w579] -> w541
              frame Default {
                n251 = Subtract(x=w554, y=w551) -> (x-y=w557:i32)
                n252 = Absolute Value(x=w557) -> (abs(x)=w555:i32)
                n253 = Not Equal To 0?(x=w555) -> (x != 0?=w556:bool)
                n254 = case shown="True" w556 {
                  tunnel: w555 -> [_ w567]
                  tunnel: [w559 w562] -> w553
                  tunnel: w552 -> [w559 w561]
                  tunnel: w551 -> [_ w560]
                  frame False {
                  }
                  frame True {
                    n255 = To Double Precision Float(number=w567) -> (double precision float=w566:dbl)
                    n256 = To Double Precision Float(number=w560) -> (double precision float=w568:dbl)
                    n257 = Divide(x=w566, y=w568) -> (x/y=w565:dbl)
                    n258 = Greater Or Equal?(x=w565, y=0.01) -> (x >= y?=w563:bool)
                    n259 = case shown="False" w563 {
                      tunnel: [w569 w572] -> w562
                      tunnel: w561 -> [w569 w570]
                      frame False {
                      }
                      frame True {
                        w571 = T13[] [enum."StopMeas"] items=["Idle", "Init", "SetInpChan", "SetSyncDivider", "SetSyncTrg", "SetSyncOffset", "SetSyncDeadTime", "SetBinning", "SetHistoOffset", "SetHistoLen", "SetStopOvl", "SetBitShift", "SetHistoAcqTime", "GetRates", "GetAllRates", "StartMeas", "StopMeas", "AbortMeas", "GetResolution", "GetHistos", "GetAllHistos", "ReadFiFo", "WriteStatus", "Resize", "EnableControls", "DisableControls", "Error", "Exit"]
                        n260 = One Button Dialog(message="Warning: Sync Rate has changed!\nTime Trace resolution has been changed accordingly.\nMeasurement is aborted.\n") -> ()  [unwired: 1 in, 1 out]
                        n261 = Build Array (concatenate)(w570, w571) -> (w572:T13[])
                      }
                    }
                  }
                }
              }
              frame -1 {
                n262 = Bundle By Name(cluster=w576, "SyncRateStart"=w575) -> (w574:T9)
              }
              frame -2 {
                n263 = Bundle By Name(cluster=w580, "SyncRateStart"=-1) -> (w579:T9)
              }
            }
          }
        }
        n264 = Bundle By Name(cluster=w519, "SyncRate"=w524) -> (w530:T9)
        n265 = Format Into String(format string="Sync Rate: %d cps\n", w524) -> (resulting string=→"SyncRate":string)  [unwired: 2 in, 1 out]
      }
      frame "GetRates" {
        # "An alternative to GetAllRates"
        n266 = Unbundle By Name(w586) -> ("Init Info.nchannels"=w591:i32, "Channels"=w587:T3[], "DevIdx"=w588:i32)
        n267 = call "MH_GetSyncRate.vi"("devidx"=w588) -> ("error out"=w590:errorcluster, "syncrate"=w584:i32)  [unwired: 8 in, 1 out]
        n268 = Format Into String(format string="Sync Rate: %d cps\n", w584) -> (resulting string=w583:string)  [unwired: 2 in, 1 out]
        n269 = local write "SyncRate"(w583) -> ()
        n270 = for {
          N: w591 -> [_]
          tunnel: w588 -> [w599]
          tunnel: [w596] -> w582 mode=indexing
          shift-right: [w598] -> w592
          shift-left: w590 -> [w600]
          tunnel: w587 -> [w595] mode=indexing
          i -> [w597]
          n271 = Unbundle By Name(w595) -> ("Enable"=w594:bool)
          n272 = case shown="True" w594 {
            tunnel: w600 -> [w601 w606]
            tunnel: w599 -> [_ w605]
            tunnel: [w601 w604] -> w598
            tunnel: w597 -> [_ w603]
            tunnel: [_ w602] -> w596
            frame False {
            }
            frame True {
              n273 = call "MH_GetCountRate.vi"("error in (no error)"=w606, "Channel"=w603, "devidx"=w605) -> ("error out"=w604:errorcluster, "rate"=w602:i32)  [unwired: 6 in, 1 out]
            }
          }
        }
        n274 = local write "CountRates"(w582) -> ()
        n275 = Bundle By Name(cluster=w586, "SyncRate"=w584) -> (w585:T9)
      }
      frame "StartMeas" {
        n276 = Bundle By Name(cluster=T8 {"Cmd"=enum."Proc", "nActual"=0, "Buffer"=[], "TickCount"=0, "Param"=0} ("MH_DataProcThread_QData"), "Cmd"=MH_DataProcThread_QCmds."Init") -> (w611:T8)
        n277 = Unbundle By Name(w609) -> ("DevIdx"=w618:i32, "AcqTime"=w614:i32)
        n278 = Enqueue Element(queue=w613, element=w611) -> ()  [unwired: 2 in, 3 out]
        n279 = Bundle By Name(cluster=w609, "SyncRateStart"=-2) -> (w608:T9)
        n280 = call "MH_StartMeas.vi"("tacq"=w614, "devidx"=w618) -> ("error out"=w619:errorcluster)  [unwired: 8 in, 1 out]
        n281 = Build Array (concatenate)(w617, MH_UIThread_Cmds."ReadFiFo") -> (w616:T13[])
      }
      frame "StopMeas" {
        n282 = Unbundle By Name(w625) -> ("Run cont."=w620:bool, "DevIdx"=w626:i32)
        n283 = call "MH_StopMeas.vi"("devidx"=w626) -> ("error out"=w627:errorcluster)  [unwired: 9 in, 1 out]
        n284 = case shown="False" w620 {
          tunnel: w625 -> [w631 w633]
          tunnel: [w630 w633] -> w624
          tunnel: [w628 w632] -> w623
          frame False {
            w628 = T13[] [enum."ReadFiFo"] items=["Idle", "Init", "SetInpChan", "SetSyncDivider", "SetSyncTrg", "SetSyncOffset", "SetSyncDeadTime", "SetBinning", "SetHistoOffset", "SetHistoLen", "SetStopOvl", "SetBitShift", "SetHistoAcqTime", "GetRates", "GetAllRates", "StartMeas", "StopMeas", "AbortMeas", "GetResolution", "GetHistos", "GetAllHistos", "ReadFiFo", "WriteStatus", "Resize", "EnableControls", "DisableControls", "Error", "Exit"]
            w629 = FALSE ("StartMeas")
            n285 = Bundle By Name(cluster=w631, "StartMeas"=w629) -> (w630:T9)
            n286 = local write "Start"(w629) -> ()
          }
          frame True {
            w632 = T13[] [enum."ReadFiFo", enum."StartMeas"] items=["Idle", "Init", "SetInpChan", "SetSyncDivider", "SetSyncTrg", "SetSyncOffset", "SetSyncDeadTime", "SetBinning", "SetHistoOffset", "SetHistoLen", "SetStopOvl", "SetBitShift", "SetHistoAcqTime", "GetRates", "GetAllRates", "StartMeas", "StopMeas", "AbortMeas", "GetResolution", "GetHistos", "GetAllHistos", "ReadFiFo", "WriteStatus", "Resize", "EnableControls", "DisableControls", "Error", "Exit"]
          }
        }
        n287 = Build Array (concatenate)(w622, w623) -> (w621:T13[])
      }
      frame "AbortMeas" {
        w635 = FALSE ("StartMeas")
        n288 = Unbundle By Name(w637) -> ("DevIdx"=w638:i32)
        n289 = call "MH_StopMeas.vi"("devidx"=w638) -> ("error out"=w639:errorcluster)  [unwired: 9 in, 1 out]
        n290 = Bundle By Name(cluster=w637, "StartMeas"=w635) -> (w636:T9)
        n291 = local write "Start"(w635) -> ()
      }
      frame "GetResolution" {
        # "Resolution in ns"
        # "Gets resolution in ps"
        # "Resolution is saved in UIThread Data cluster in ns"
        n292 = Unbundle By Name(w648) -> ("DevIdx"=w650:i32)
        n293 = call "MH_GetResolution.vi"("devidx"=w650) -> ("error out"=w649:errorcluster, "resolution"=w646:dbl)  [unwired: 8 in, 1 out]
        n294 = Divide(x=w646, y=1000.0) -> (x/y=w642:dbl)
        n295 = Bundle By Name(cluster=w648, "Resolution"=w642) -> (w647:T9)
        n296 = Bundle By Name(cluster=T6 {"Histos"=[], "Cmd"=enum."_none_", "TimeTrace"=[], "Bin"=0, "Total bin"=0, "Status"="", "Resol"=0.0, "DeltaT"=0.0, "nChannels"=0} ("MH_GUIThread_QData"), "Resol"=w642, "Cmd"=MH_VisThread_QCmds."Resol") -> (w640:T6)
        n297 = Enqueue Element(queue=w644, element=w640) -> ()  [unwired: 2 in, 3 out]
      }
      frame "ReadFiFo" {
        w660 = 2  # FLAG_FIFOFULL
        # "Reads photon records from HW and transferes them to DataProcThread via Queue."
        n298 = Unbundle By Name(w662) -> ("DevIdx"=w656:i32)
        n299 = call "MH_GetFlags.vi"("devidx"=w656) -> ("error out"=w658:errorcluster, "flags"=w659:i32)  [unwired: 8 in, 1 out]
        n300 = And(x=w659, y=w660) -> (x .and. y?=w661:i32)
        n301 = Not Equal To 0?(x=w661) -> (x != 0?=w655:bool)
        "OverRun" <- w655
        n302 = case shown="False" w655 {
          tunnel: w658 -> [w672 w675]
          tunnel: [w671 w675] -> w657
          tunnel: w656 -> [w664 _]
          tunnel: w654 -> [w670 _]
          tunnel: w653 -> [w669 _]
          tunnel: [w669 w673] -> w652
          frame False {
            n303 = call "MH_ReadFiFo.vi"("error in (no error)"=w672, "devidx"=w664) -> ("error out"=w671:errorcluster, "nactual"=w663:i32, "buffer"=w667:u32[])  [unwired: 6 in, 1 out]
            n304 = Bundle By Name(cluster=T8 {"Cmd"=enum."Proc", "nActual"=0, "Buffer"=[], "TickCount"=0, "Param"=0} ("MH_DataProcThread_QData"), "Buffer"=w667, "nActual"=w663, "Cmd"=MH_DataProcThread_QCmds."Proc") -> (w665:T8)
            n305 = Enqueue Element(queue=w670, element=w665) -> ()  [unwired: 2 in, 3 out]
          }
          frame True {
            n306 = Build Array(MH_UIThread_Cmds."AbortMeas") -> (w673:T13[])
          }
        }
      }
      frame "WriteStatus" {
        n307 = Unbundle By Name(w677) -> ("Status"=→"Status":string)
      }
      frame "Resize" {
        n308 = property on="Pane 3" class="Pane"() -> ("Width"=w684:u32)  [unwired: 2 in, 2 out]
        n309 = Subtract(x=w684, y=i16 100 ("b")) -> (x-y=w690:u32)
        n310 = Unbundle By Name(w679) -> ("Init Info.nchannels"=w687:i32)
        n311 = Quotient & Remainder(x=w690, y=i16 99 ("m")) -> (floor(x/y)=w689:u32)  [unwired: 1 out]
        n312 = In Range and Coerce(upper limit=w687, x=w689, lower limit=4) -> (coerced(x)=w688:u32)  [unwired: 1 out]
        n313 = Equal?(x=w687, y=w688) -> (x = y?=w686:bool)
        n314 = Not(x=w686) -> (.not. x?=w685:bool)
        n315 = property on="Channels" class="Arr (strict)"("HorizScroll"=w685, "Number of Columns"=w688, "Index Values"=u32[] [0]) -> ()  [unwired: 2 in, 2 out]
      }
      frame "EnableControls" {
        n316 = property class="VI"() -> ("Panel"=w695:refnum<vi>)  [unwired: 2 in, 2 out]
        n317 = property class="Pnl"(reference=w695) -> ("Controls[]"=w694:refnum<vi>[])  [unwired: 1 in, 2 out]
        n318 = property class="Pnl"(reference=w695) -> ("Decos[]"=w696:refnum<vi>[])  [unwired: 1 in, 2 out]
        n319 = for {
          tunnel: w696 -> [w700] mode=indexing
          tunnel: TRUE -> [w699]
          n320 = property class="Decor"(reference=w700, "Visible"=w699) -> ()  [unwired: 1 in, 2 out]
        }
        n321 = for {
          tunnel: w694 -> [w703] mode=indexing
          tunnel: T14."Enabled" ("Disabled") -> [w702]
          tunnel: [w701] -> _
          n322 = property class="Ctl"(reference=w703, "DisabledEnum"=w702) -> (error out=w701:errorcluster)  [unwired: 1 in, 1 out]
        }
      }
      frame "DisableControls" {
        n323 = property class="VI"() -> ("Panel"=w707:refnum<vi>)  [unwired: 2 in, 2 out]
        n324 = property class="Pnl"(reference=w707) -> ("Controls[]"=w706:refnum<vi>[])  [unwired: 1 in, 2 out]
        n325 = property class="Pnl"(reference=w707) -> ("Decos[]"=w708:refnum<vi>[])  [unwired: 1 in, 2 out]
        n326 = for {
          tunnel: w708 -> [w712] mode=indexing
          tunnel: FALSE -> [w711]
          n327 = property class="Decor"(reference=w712, "Visible"=w711) -> ()  [unwired: 1 in, 2 out]
        }
        n328 = for {
          tunnel: w706 -> [w715] mode=indexing
          tunnel: T14."Disabled and Grayed Out" ("Disabled") -> [w714]
          tunnel: [w713] -> _
          n329 = property class="Ctl"(reference=w715, "DisabledEnum"=w714) -> (error out=w713:errorcluster)  [unwired: 1 in, 1 out]
        }
      }
      frame "Error" {
        w716 = T13[] [enum."Exit"] items=["Idle", "Init", "SetInpChan", "SetSyncDivider", "SetSyncTrg", "SetSyncOffset", "SetSyncDeadTime", "SetBinning", "SetHistoOffset", "SetHistoLen", "SetStopOvl", "SetBitShift", "SetHistoAcqTime", "GetRates", "GetAllRates", "StartMeas", "StopMeas", "AbortMeas", "GetResolution", "GetHistos", "GetAllHistos", "ReadFiFo", "WriteStatus", "Resize", "EnableControls", "DisableControls", "Error", "Exit"]
        w719 = T18 1 items=["no dialog", "OK message", "continue or stop message", "OK message + warnings", "continue/stop + warnings"] ("type of dialog (OK msg:1)")
        # "Error case: If an error occures the user is informed and the programm terminates. Add your own code to handle error events (e.g. exception lists, etc.)"
        n330 = call <vilib>:"Simple Error Handler.vi"("type of dialog (OK msg:1)"=w719, "error in (no error)"=w718) -> ()  [unwired: 3 in, 5 out]
      }
      frame "Exit" {
        n331 = Release Queue(queue=w721) -> ()  [unwired: 2 in, 3 out]
        n332 = Release Queue(queue=w720) -> ()  [unwired: 2 in, 3 out]
        n333 = Unbundle By Name(w725) -> ("DevIdx"=w724:i32)
        n334 = call "MH_CloseDevice.vi"("devidx"=w724) -> ("error out"=w723:errorcluster)  [unwired: 9 in, 1 out]
      }
    }
    n335 = call "MH_EnQError.vi"("error in (no error)"=w24, "Cmds_in"=w22) -> ("error out"=w23:errorcluster, "Cmds_out"=w21:T13[])  [unwired: 8 in]
  }
  n336 = call "MH_DataProcThread.vi"("MH_VisThread_QRef"=w7, "MH_DataProcThread_QRef"=w1) -> ()  [unwired: 10 in]
  n337 = while {
    tunnel: w7 -> [w734]
    shift-right: [w730] -> _
    shift-left: T5 {"Resol"=0.0, "DeltaT"=0.0, "NumChannels"=0} -> [w731]
    tunnel: w1 -> [w729]
    stop <- w727 stop-if-true
    # "VisualizationThread"
    n338 = Dequeue Element(queue=w734, timeout in ms (-1)=100) -> (element=w732:T6, error out=w727:errorcluster)  [unwired: 1 in, 2 out]
    n339 = Unbundle By Name(w732) -> ("Cmd"=w733:T7)
    n340 = case shown="\"TTrace\"" w733 {
      tunnel: w732 -> [_ w747 w749 w761 w769 w773 w777]
      tunnel: w731 -> [w737 w745 w751 w753 w768 w772 w776]
      tunnel: [w737 w745 w750 w753 w768 w771 w775] -> w730
      tunnel: w729 -> [w736 _ _ _ w765 _ _]
      tunnel: w727 -> [w735 _ _ _ _ _ _]
      frame "_none_", Default {
        n341 = case shown="No Error" w735 {
          tunnel: w736 -> [w741 _]
          frame No Error {
            n342 = Get Queue Status(queue=w741) -> (# elements in queue=w739:i32)  [unwired: 2 in, 7 out]
            n343 = Format Into String(format string="Elements in Q: %d", w739) -> (resulting string=w738:string)  [unwired: 2 in, 1 out]
            n344 = local write "Status"(w738) -> ()
          }
          frame Error {
          }
        }
      }
      frame "Histo" {
        n345 = Unbundle By Name(w747) -> ("Histos"=w742:u32[][])
        n346 = Unbundle By Name(w745) -> ("Resol"=w744:dbl)
        n347 = Bundle(0.0, "Resol"=w744, "Histos"=w742) -> (→"HistoGraph":cluster{dbl, "Resol":dbl, "Histos":u32[][]})  [unwired: 1 in]
      }
      frame "nChannels" {
        n348 = Unbundle By Name(w749) -> ("nChannels"=w748:i32)
        n349 = Bundle By Name(cluster=w751, "NumChannels"=w748) -> (w750:T5)
      }
      frame "TTrace" {
        n350 = Unbundle By Name(w761) -> ("Total bin"=w760:u64, "Bin"=w759:i32, "TimeTrace"=w758:u32[][])
        n351 = Unbundle By Name(w753) -> ("DeltaT"=w752:dbl)
        n352 = call "MH_TTraceToGraph.vi"("DeltaT"=w752, "TimeTrace"=w758, "Bin"=w759, "Total bin"=w760) -> ("TimeTrace_out"=w755:u32[][], "dt"=w756:dbl, "T0"=w757:dbl)  [unwired: 5 in]
        n353 = Bundle("T0"=w757, "dt"=w756, "TimeTrace_out"=w755) -> (→"TTraceGraph":T19)  [unwired: 1 in]
      }
      frame "Status" {
        n354 = Unbundle By Name(w769) -> ("Status"=w766:string)
        n355 = Get Queue Status(queue=w765) -> (# elements in queue=w764:i32)  [unwired: 2 in, 7 out]
        n356 = Format Into String(format string="\t\tElements in Q: %d", w764) -> (resulting string=w762:string)  [unwired: 2 in, 1 out]
        n357 = Concatenate Strings(w766, w762) -> (w767:string)
        n358 = local write "Status"(w767) -> ()
      }
      frame "DeltaT" {
        n359 = Unbundle By Name(w773) -> ("DeltaT"=w770:dbl)
        n360 = Bundle By Name(cluster=w772, "DeltaT"=w770) -> (w771:T5)
      }
      frame "Resol" {
        n361 = Unbundle By Name(w777) -> ("Resol"=w774:dbl)
        n362 = Bundle By Name(cluster=w776, "Resol"=w774) -> (w775:T5)
      }
    }
  }
